vi "Run.vi"(8 "error in (no error)":errorcluster, 9 "Time Ratio used":dbl, 10 "Maze (0: Empty, -1: Enemy. >0: Teammate":i32[][](array[numeric]), 11 "Line Dancer in":refnum<class "Line Dancer.lvclass">) -> (0 "error out":errorcluster, 1 "Direction":T1, 2 "Action":T2, 3 "Line Dancer out":refnum<class "Line Dancer.lvclass">, 4 "Replicated":refnum<class "Square.lvclass">)   [LabVIEW 2015, in "Line Dancer.lvclass"]
uses:
  Line Dancer.lvclass
  Type Defs/Action Enum.ctl
  Type Defs/Direction Enum.ctl
  Square/Square.lvclass
  Line Dancer.lvclass/Line Dancer.ctl
  Line Dancer Type.ctl
  SubVIs/Read-Only Globals.vi
  Type Defs/SB Type Defs.lvlib
  Common/Common.lvlib
panel:
  # "NOTICE - YOU MUST NOT REMOVE THIS NOTICE. PER THE FOLLOWING LICENSE, YOU MAY REPRODUCE THIS SOFTWARE PROVIDED YOU FOLLOW THE TERMS\nOF THE LICENSE.\n\n---BEGIN BSD LICENSE (http://opensource.org/licenses/BSD-2-Clause)---\nCopyright (c) 2015, Endigit, Inc. <robert@endigit.com>\nAll rights reserved.\n\nRedistribution and use in source and binary forms, with or without modification, are permitted provided that the following conditions are met:\n\n1. Redistributions of source code must retain the above copyright notice, this list of conditions and the following disclaimer.\n\n2. Redistributions in binary form must reproduce the above copyright notice, this list of conditions and the following disclaimer in the documentation and/or other \nmaterials provided with the distribution.\n\nTHIS SOFTWARE IS PROVIDED BY THE COPYRIGHT HOLDERS AND CONTRIBUTORS \"AS IS\" AND ANY EXPRESS OR IMPLIED WARRANTIES, INCLUDING, BUT NOT \nLIMITED TO, THE IMPLIED WARRANTIES OF MERCHANTABILITY AND FITNESS FOR A PARTICULAR PURPOSE ARE DISCLAIMED. IN NO EVENT SHALL THE COPYRIGHT \nHOLDER OR CONTRIBUTORS BE LIABLE FOR ANY DIRECT, INDIRECT, INCIDENTAL, SPECIAL, EXEMPLARY, OR CONSEQUENTIAL DAMAGES (INCLUDING, BUT NOT \nLIMITED TO, PROCUREMENT OF SUBSTITUTE GOODS OR SERVICES; LOSS OF USE, DATA, OR PROFITS; OR BUSINESS INTERRUPTION) HOWEVER CAUSED AND ON \nANY THEORY OF LIABILITY, WHETHER IN CONTRACT, STRICT LIABILITY, OR TORT (INCLUDING NEGLIGENCE OR OTHERWISE) ARISING IN ANY WAY OUT OF THE USE \nOF THIS SOFTWARE, EVEN IF ADVISED OF THE POSSIBILITY OF SUCH DAMAGE.\n---END BSD LICENSE---"
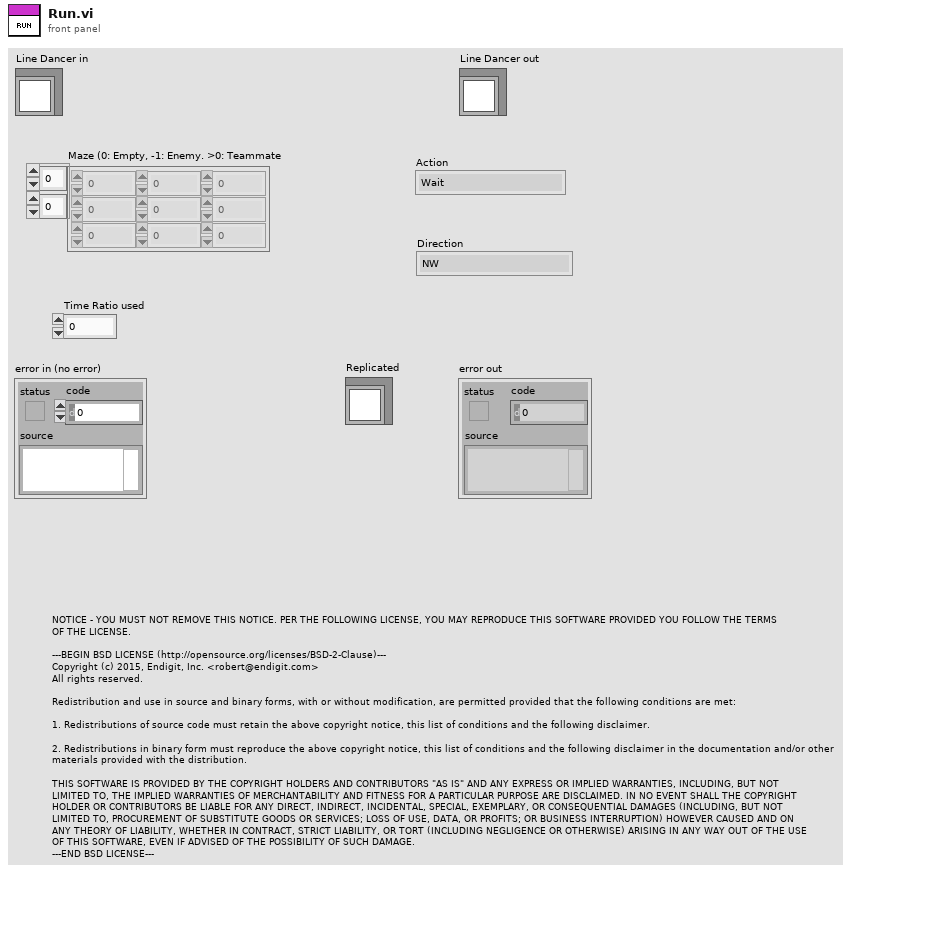
[diagram p1: front panel]
types:
  T1 = typedef "SB Type Defs.lvlib/Direction Enum.ctl" = enum16{"NW", "N", "NE", "E", "SE", "S", "SW", "W"}
  T2 = typedef "SB Type Defs.lvlib/Action Enum.ctl" = enum16{"Wait", "Move", "Attack", "Replicate"}
  T3 = typedef "Line Dancer.lvclass/Line Dancer Type.ctl" = enum16{"Top", "Bottom", "Start"}
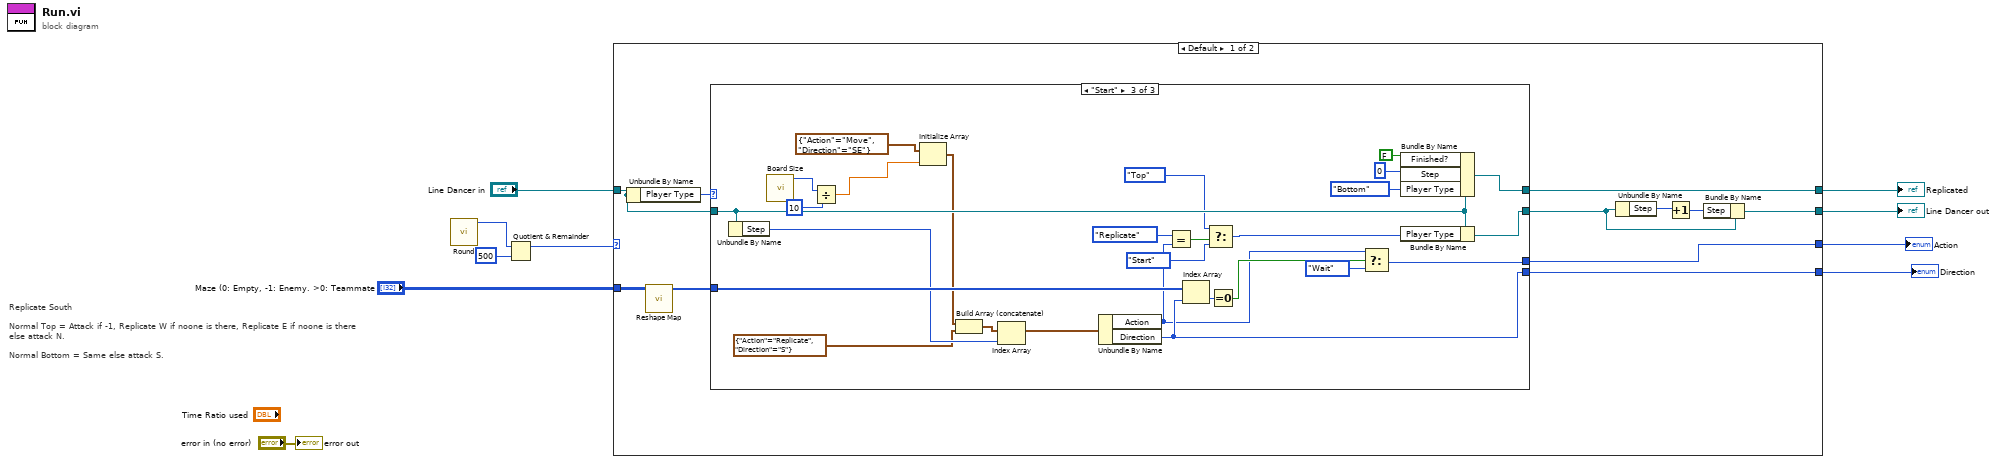
[diagram p0: block diagram]
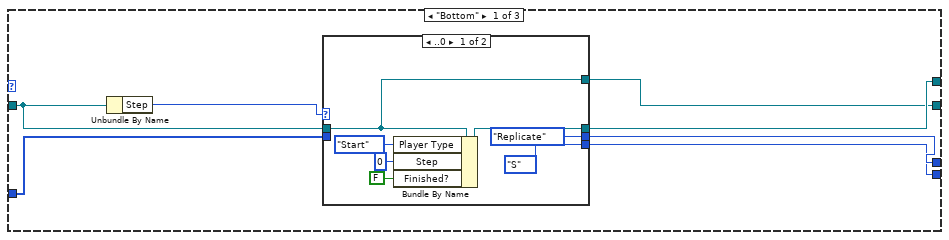
[diagram p2: hidden frame]
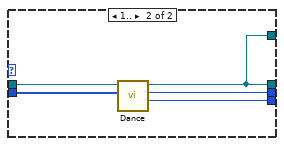
[diagram p3: hidden frame]
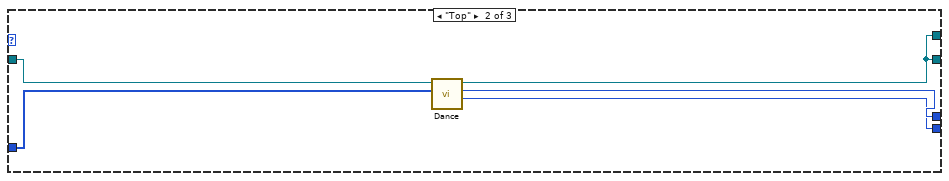
[diagram p4: hidden frame]
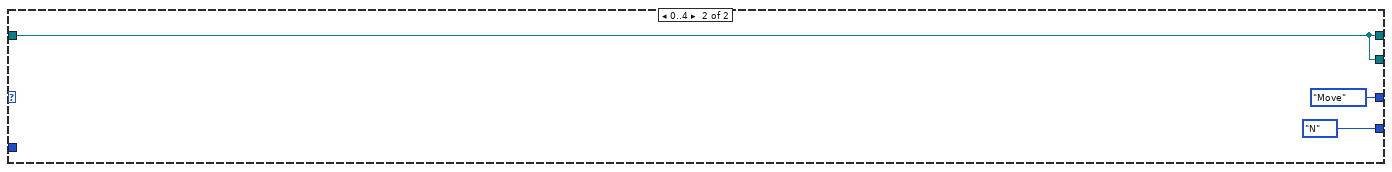
[diagram p5: hidden frame]
diagram:
  # "Replicate South\n\nNormal Top = Attack if -1, Replicate W if noone is there, Replicate E if noone is there\nelse attack N.\n\nNormal Bottom = Same else attack S."
  n1 = call "Round.vi"() -> ("Round"=w3:i32)  [unwired: 11 in]
  n2 = Quotient & Remainder(x=w3, y=500) -> (x-y*floor(x/y)=w1:i32)  [unwired: 1 out]
  n3 = case shown="Default" w1 {
    tunnel: [w21 Action_Enum."Move" ("f")] -> w9
    tunnel: [w20 Direction_Enum."N" ("Direction")] -> w8
    tunnel: "Maze (0: Empty, -1: Enemy. >0: Teammate" -> [w19 _]
    tunnel: "Line Dancer in" -> [w16 w75]
    tunnel: [w12 w75] -> w5
    tunnel: [w11 w75] -> w4
    frame Default {
      n4 = Unbundle By Name(w16) -> ("Player Type"=w17:T3)
      n5 = call "Reshape Map.vi"("Maze (0: Empty, -1: Enemy. >0: Teammate"=w19) -> ("Map"=w18:i32[])  [unwired: 9 in, 1 out]
      n6 = case shown="\"Start\"" w17 {
        tunnel: [w28 w45 w62] -> w21
        tunnel: [w27 w44 w67] -> w20
        tunnel: w18 -> [w26 w43 w68]
        tunnel: [w25 w41 w71] -> w11
        tunnel: [w22 w41 w70] -> w13
        tunnel: w16 -> [w24 w42 w65]
        frame "Bottom" {
          n7 = Unbundle By Name(w24) -> ("Step"=w23:i32)
          n8 = case shown="..0" w23 {
            tunnel: [Action_Enum."Replicate" ("Action") w40] -> w28
            tunnel: [Direction_Enum."S" ("Direction") w39] -> w27
            tunnel: w26 -> [_ w38]
            tunnel: [w33 w36] -> w25
            tunnel: w24 -> [w29 w37]
            tunnel: [w29 w36] -> w22
            frame ..0 {
              n9 = Bundle By Name(cluster=w29, "Player Type"=Line_Dancer_Type."Start", "Step"=0, "Finished?"=FALSE) -> (w33:refnum<class "Line Dancer.lvclass">)
            }
            frame 1.. {
              n10 = call "Dance.vi"("Map"=w38, "Line Dancer in"=w37) -> ("index of element"=w39:i32, "Action"=w40:T2, "Line Dancer out"=w36:refnum<class "Line Dancer.lvclass">)  [unwired: 7 in]
            }
          }
        }
        frame "Top" {
          n11 = call "Dance.vi"("Map"=w43, "Line Dancer in"=w42) -> ("index of element"=w44:i32, "Action"=w45:T2, "Line Dancer out"=w41:refnum<class "Line Dancer.lvclass">)  [unwired: 7 in]
        }
        frame "Start" {
          n12 = Unbundle By Name(w65) -> ("Step"=w63:i32)
          n13 = call "Board Size.vi"() -> ("Board Size"=w48:i32)  [unwired: 11 in]
          n14 = Divide(x=w48, y=10) -> (x/y=w46:dbl)
          n15 = Initialize Array(cluster{"Action":T2, "Direction":T1} {"Action"=enum."Move", "Direction"=enum."SE"}, w46) -> (w49:cluster{"Action":T2, "Direction":T1}[])
          n16 = Build Array (concatenate)(w49, cluster{"Action":T2, "Direction":T1} {"Action"=enum."Replicate", "Direction"=enum."S"}) -> (w51:cluster{"Action":T2, "Direction":T1}[])
          n17 = Index Array(array=w51, index=w63) -> (element=w66:cluster{"Action":T2, "Direction":T1})
          n18 = Unbundle By Name(w66) -> ("Action"=w58:T2, "Direction"=w67:T1)
          n19 = Equal?(x=Action_Enum."Replicate", y=w58) -> (x = y?=w59:bool)
          n20 = Index Array(array=w68, index=w67) -> (element=w64:i32)
          n21 = Select(t=Line_Dancer_Type."Top" ("Player Type"), s=w59, f=Line_Dancer_Type."Start" ("Player Type")) -> (s? t:f=w54:T3)
          n22 = Equal To 0?(x=w64) -> (x = 0?=w61:bool)
          n23 = Select(t=w58, s=w61, f=Action_Enum."Wait") -> (s? t:f=w62:T2)
          n24 = Bundle By Name(cluster=w65, "Finished?"=FALSE, "Step"=0, "Player Type"=Line_Dancer_Type."Bottom") -> (w71:refnum<class "Line Dancer.lvclass">)
          n25 = Bundle By Name(cluster=w65, "Player Type"=w54) -> (w70:refnum<class "Line Dancer.lvclass">)
        }
      }
      n26 = Unbundle By Name(w13) -> ("Step"=w15:i32)
      n27 = Increment(x=w15) -> (x+1=w14:i32)
      n28 = Bundle By Name(cluster=w13, "Step"=w14) -> (w12:refnum<class "Line Dancer.lvclass">)
    }
    frame 0..4 {
    }
  }
  "Line Dancer out" <- w5
  "Action" <- w9
  "Direction" <- w8
  "Replicated" <- w4
  "error out" <- "error in (no error)"
